vi "Load Profile.vi"(0 "F4T in":refnum<class "F4T.lvclass">, 5 "Profile Number":u32=1 min=1 step=1, 7 "Profile Name":string, 9 "Profile Steps":string[][](array[string]), 11 "error in (no error)":errorcluster) -> (4 "F4T out":refnum<class "F4T.lvclass">, 15 "error out":errorcluster)   [LabVIEW 2018, in "F4T.lvlib" / "F4T.lvclass"]
doc: "This Override is used to load a Profile to the Temp Chamber. It requires a Profile Number and the profile information is passed as a 2D atring array."
uses:
  F4T.lvclass
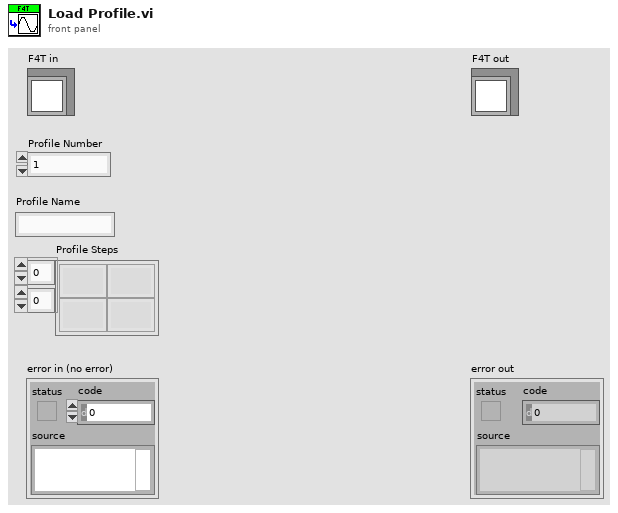
[diagram p1: front panel]
types:
  T1 = typedef "F4T.lvlib/F4T.lvclass/Command Data.ctl" = cluster{"ParameterID":u32, "InstanceId":u32, "Value":string}
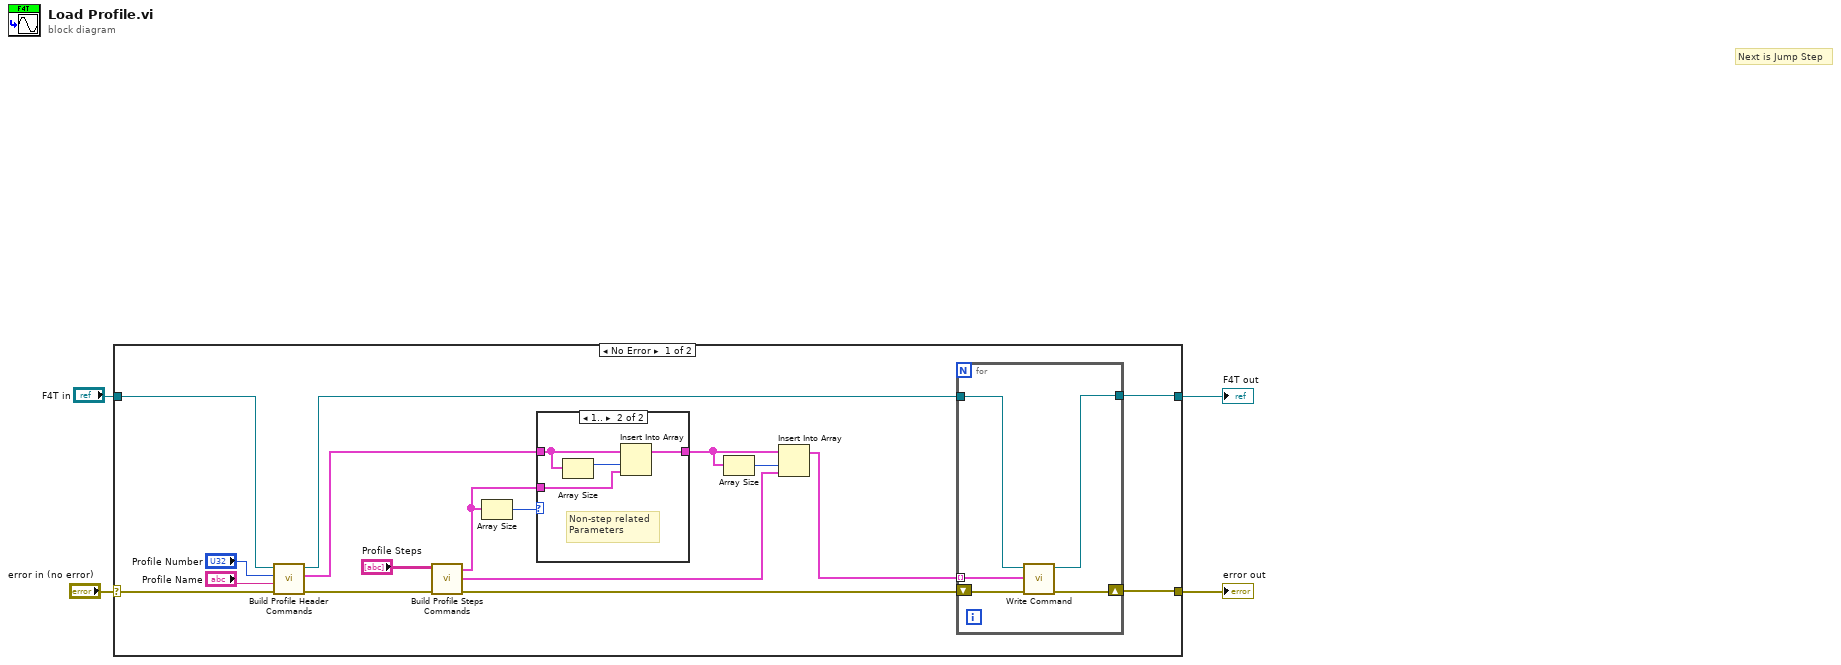
[diagram p0: block diagram]
diagram:
  # "Next is Jump Step"
  n1 = case shown="No Error" "error in (no error)" {
    selector: "error in (no error)" -> [w21 w33]
    tunnel: "F4T in" -> [w10 w32]
    tunnel: [w13 w33] -> w2
    tunnel: [w14 w32] -> w1
    frame No Error {
      n2 = call "Build Profile Header Commands.vi"("error in"=w21, "Profile Name"="Profile Name", "Profile Number"="Profile Number", "F4T in"=w10) -> ("error out"=w20:errorcluster, "Profile Header Commands"=w7:T1[], "F4T out"=w9:refnum<class "F4T.lvclass">)  [unwired: 5 in]
      n3 = call "Build Profile Steps Commands.vi"("error in"=w20, "Profile Steps"="Profile Steps") -> ("error out"=w15:errorcluster, "Param Only Commands"=w6:T1[], "Profile Steps Commands"=w17:T1[])  [unwired: 7 in]
      n4 = Array Size(array=w6) -> (size(s)=w8:i32)
      n5 = case shown="1.." w8 {
        tunnel: w7 -> [w22 w26]
        tunnel: w6 -> [_ w24]
        tunnel: [w22 w23] -> w5
        frame 0, Default {
        }
        frame 1.. {
          # "Non-step related\nParameters"
          n6 = Array Size(array=w26) -> (size(s)=w25:i32)
          n7 = Insert Into Array(array=w26, index=w25, new element=w24) -> (w23:T1[])
        }
      }
      n8 = Array Size(array=w5) -> (size(s)=w18:i32)
      n9 = Insert Into Array(array=w5, index=w18, new element=w17) -> (w16:T1[])
      n10 = for {
        tunnel: w16 -> [w30] mode=indexing
        tunnel: w9 -> [w29]
        shift-right: [w28] -> w13
        shift-left: w15 -> [w31]
        tunnel: [w27] -> w14
        n11 = call "Write Command.vi"("error in (no error)"=w31, "Command Data"=w30, "F4T in"=w29) -> ("error out"=w28:errorcluster, "F4T out"=w27:refnum<class "F4T.lvclass">)  [unwired: 7 in]
      }
    }
    frame Error {
    }
  }
  "error out" <- w2
  "F4T out" <- w1
